vi "SciScan HYPERSCOPE.vi"() -> ()   [LabVIEW 2012]
uses:
  GFG/GFG Translator Wrapper/GFGTranslator_Action.ctl
  GFG/GFG Translator Wrapper/GFGTranslator_Datatype.ctl
  <vilib>/Utility/config.llb/Read Key (String).vi
  <vilib>/Utility/config.llb/NI_LVConfig.lvlib
panel:
  in  "Quit Button":bool
  in  "Imaging Path Reso":bool
  in  "Imaging Path Galvo":bool
  in  "Stimulation Path Galvo":bool
  # "HyperScope Main Control"
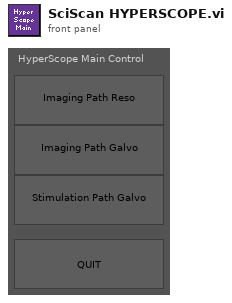
[diagram p1: front panel]
types:
  T1 = enum8{"Enabled", "Disabled", "Disabled and Grayed Out"}
  T2 = typedef "NI_LVConfig.lvlib/Config Data RefNum.ctl" = refnum<k1>
  T3 = enum32{"Invalid", "Standard", "Closed", "Hidden", "Minimized", "Maximized"}
  T4 = typedef "GFGTranslator_Datatype.ctl" = enum16{"String", "Path (String)", "Numeric", "Boolean", "Set_BoolRef (use boolean data)", "Get_Variant", "Get_2DArray (I16)", "Get_Image_2DArray (I16)", "Get_Version (String)", "Get_All GFG variables (String)"}
  T5 = typedef "GFGTranslator_Action.ctl" = enum16{"Get", "Set"}
  T6 = enum16{"Standalone Galvo", "Imaging Galvo", "Photostimulation Galvo"}
  T7 = typedef "GFGTranslator_errors.ctl" = enum16{"Success", "SciScan Not Running", "No Get Method for Selected Datatype", "No Set Method for Selected Datatype", "Variable Not Found", "Unexpected Datatype", "Data Out of Range"}
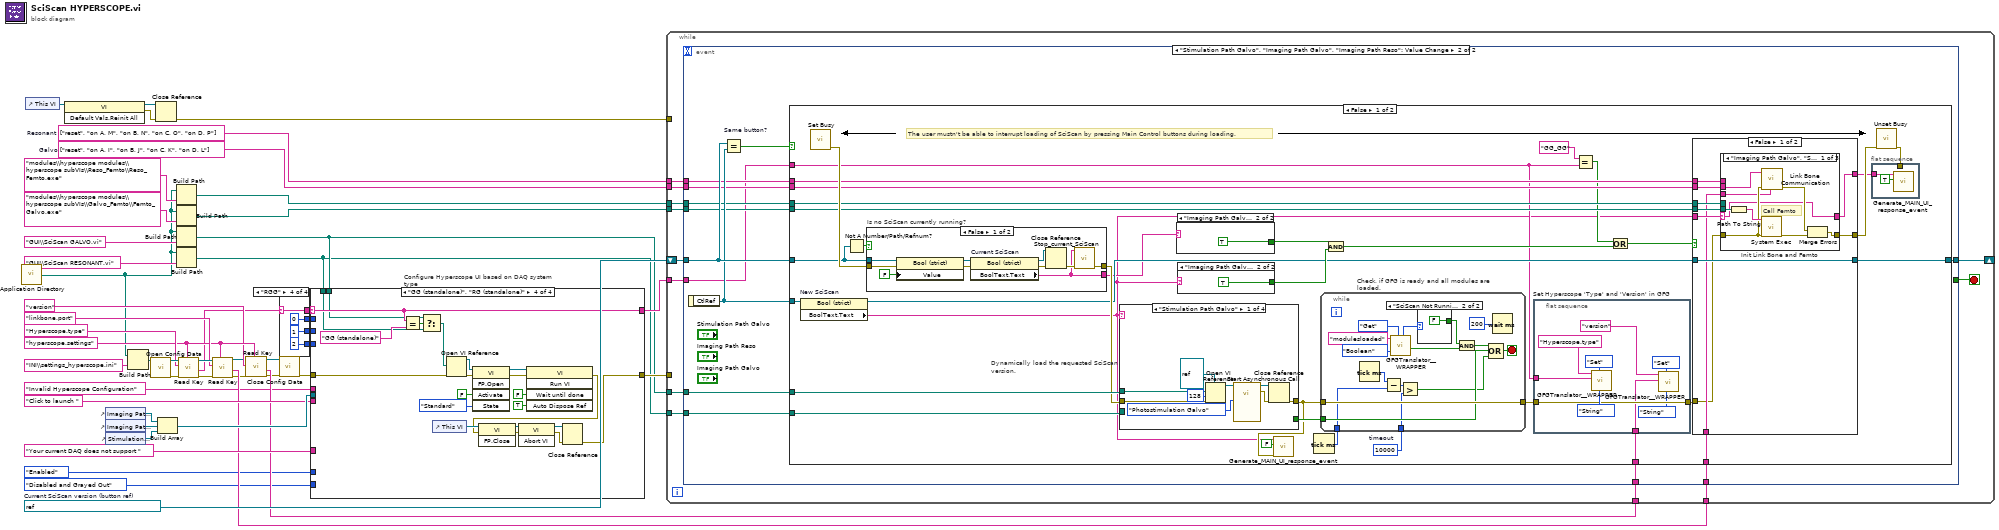
[diagram p0: block diagram]
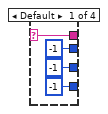
[diagram p2: hidden frame]
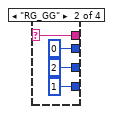
[diagram p3: hidden frame]
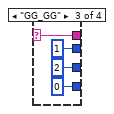
[diagram p4: hidden frame]
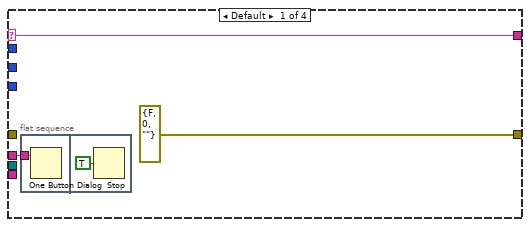
[diagram p5: hidden frame]
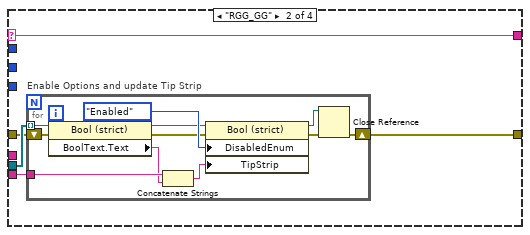
[diagram p6: hidden frame]
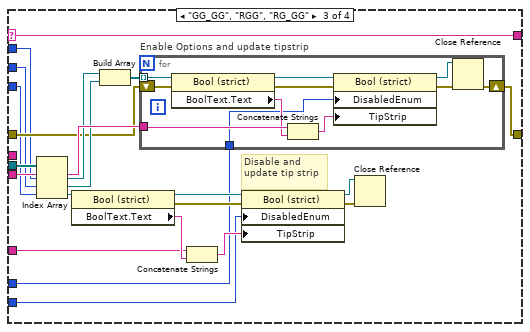
[diagram p7: hidden frame]
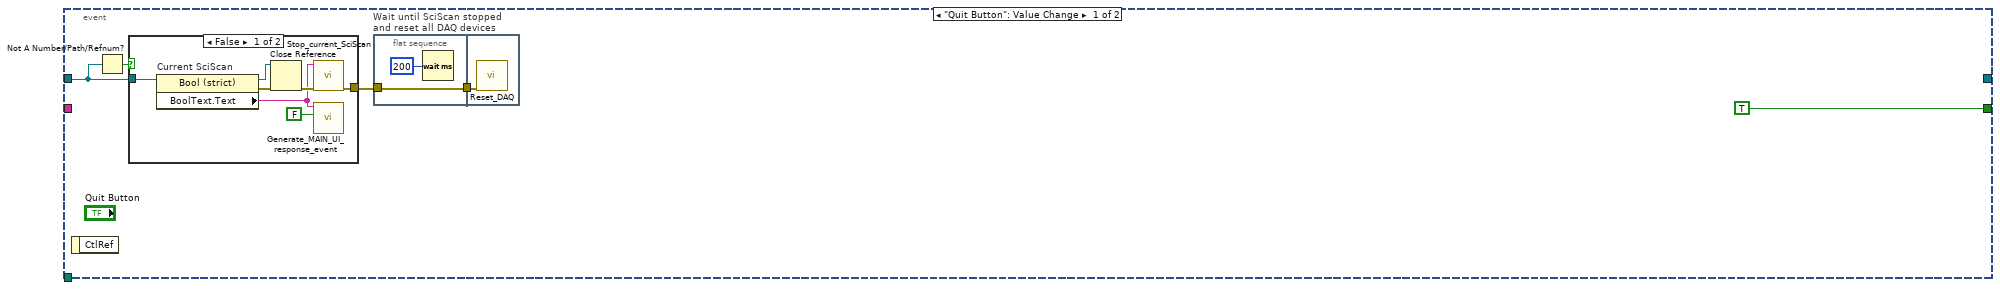
[diagram p8: hidden frame]
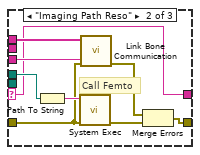
[diagram p12: hidden frame]
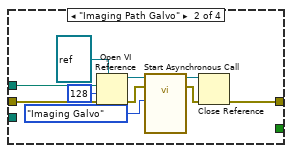
[diagram p15: hidden frame]
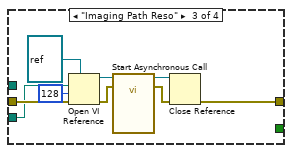
[diagram p16: hidden frame]
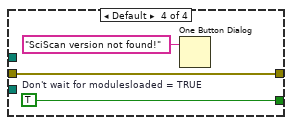
[diagram p17: hidden frame]
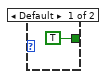
[diagram p18: hidden frame]
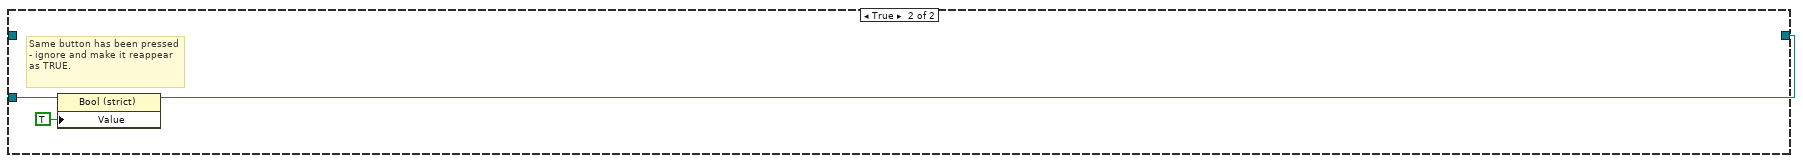
[diagram p20: hidden frame]
diagram:
  w18 = "hyperscope.settings" ("section")
  w40 = string[] ["reset", "on A, I", "on B, J", "on C, K", "on D, L"]  # Galvo
  w41 = string[] ["reset", "on A, M", "on B, N", "on C, O", "on D, P"]  # Resonant
  w42 = refnum<k0> refnum  # Current SciScan version (button ref)
  n1 = call <vilib>:"Application Directory.vi"() -> ("Application Directory"=w3:path)
  n2 = control-ref of="This VI"() -> (w48:refnum<vi>)
  n3 = invoke class="VI" method="Default Vals.Reinit All"(reference=w48) -> (reference out=w46:refnum<vi>, error out=w47:errorcluster)  [unwired: 2 in, 1 out]
  n4 = control-ref of="Imaging Path Reso"() -> (w30:refnum<vi>)
  n5 = control-ref of="Imaging Path Galvo"() -> (w29:refnum<vi>)
  n6 = control-ref of="Stimulation Path Galvo"() -> (w28:refnum<vi>)
  n7 = Build Path(base path=w3, name or relative path="INI\\settings_hyperscope.ini") -> (appended path=w34:path)
  n8 = call <vilib>:"Open Config Data.vi"("configuration file path"=w34) -> ("error out"=w33:errorcluster, "refnum"=w32:T2)  [unwired: 8 in, 1 out]
  n9 = Close Reference(reference=w46, error in (no error)=w47) -> (error out=w45:errorcluster)
  n10 = Build Array(w30, w29, w28) -> (w27:refnum<vi>[])
  n11 = Build Path(base path=w3, name or relative path="modules\\hyperscope modules\\hyperscope subVIs\\Reso_Femto\\Reso_Femto.exe") -> (appended path=w38:path)
  n12 = Build Path(base path=w3, name or relative path="modules\\hyperscope modules\\hyperscope subVIs\\Galvo_Femto\\Femto_Galvo.exe") -> (appended path=w39:path)
  n13 = Build Path(base path=w3, name or relative path="GUI\\SciScan GALVO.vi") -> (appended path=w2:path)
  n14 = Build Path(base path=w3, name or relative path="GUI\\SciScan RESONANT.vi") -> (appended path=w1:path)
  n15 = call-poly <vilib>:"Read Key.vi"("section"=w18, "error in (no error)"=w33, "key"="Hyperscope.type", "refnum"=w32) -> ("error out"=w19:errorcluster, "value"=w9:string, "refnum out"=w22:T2)  [unwired: 4 in, 1 out]
  n16 = call-poly <vilib>:"Read Key.vi"("section"=w18, "error in (no error)"=w19, "key"="linkbone.port", "refnum"=w22) -> ("error out"=w13:errorcluster, "value"=w20:string, "refnum out"=w15:T2)  [unwired: 4 in, 1 out]
  n17 = call-poly <vilib>:"Read Key.vi"("section"=w18, "key"="version", "refnum"=w15) -> ("value"=w16:string, "refnum out"=w14:T2)  [unwired: 5 in, 2 out]
  n18 = case shown="\"RGG\"" w9 {
    selector: w9 -> [w52 w53 w60 w64]
    tunnel: [w52 w53 w60 w64] -> w8
    tunnel: [-1 ("index") 0 ("index") 1 ("index") 0 ("index")] -> w7
    tunnel: [-1 ("index") 2 ("index") 2 ("index") 1 ("index")] -> w6
    tunnel: [-1 ("index") 1 ("index") 0 ("index") 2 ("index")] -> w5
    frame Default {
    }
    frame "RG_GG" {
    }
    frame "GG_GG" {
    }
    frame "RGG" {
    }
  }
  n19 = call <vilib>:"Close Config Data.vi"("error in (no error)"=w13, "refnum"=w14) -> ("error out"=w12:errorcluster)  [unwired: 8 in, 1 out]
  n20 = case "Configure Hyperscope UI based on DAQ system type" shown="\"GG (standalone)\", \"RG (standalone)\"" w8 {
    selector: w8 -> [w67 w71 w92 w135]
    tunnel: w27 -> [_ w74 w97 _]
    tunnel: "Click to launch " ("section") -> [_ w73 w106 _]
    tunnel: [errorcluster {"status"=FALSE, "code"=0, "source"=""} ("error out") w72 w105 w118] -> w25
    tunnel: "Your current DAQ does not support " ("section") -> [_ _ w93 _]
    tunnel: [w67 w71 w92 w135] -> w23
    tunnel: w12 -> [_ w70 w91 w139]
    tunnel: T1."Disabled and Grayed Out" ("Disabled") -> [_ _ w90 _]
    tunnel: T1."Enabled" ("Disabled") -> [_ _ w89 _]
    tunnel: w7 -> [_ _ w88 _]
    tunnel: w6 -> [_ _ w87 _]
    tunnel: w5 -> [_ _ w86 _]
    tunnel: "Invalid Hyperscope Configuration" ("message") -> [w66 _ _ _]
    tunnel: w2 -> [_ _ _ w132]
    tunnel: w1 -> [_ _ _ w131]
    frame Default {
      n21 = flat-sequence {
        tunnel: w66 -> [w68]
        frame #0 {
          n22 = One Button Dialog(message=w68) -> ()  [unwired: 1 in, 1 out]
        }
        frame #1 {
          n23 = Stop(stop? (T)=TRUE) -> ()
        }
      }
    }
    frame "RGG_GG" {
      n24 = for "Enable Options and update Tip Strip" {
        tunnel: w74 -> [w82] mode=indexing
        tunnel: w73 -> [w79]
        shift-right: [w76] -> w72
        shift-left: w70 -> [w75]
        n25 = property class="Bool (strict)"(reference=w82, error in=w75) -> (reference out=w81:refnum<vi>, error out=w80:errorcluster, "BoolText.Text"=w78:string)
        n26 = Concatenate Strings(w79, w78) -> (w77:string)
        n27 = property class="Bool (strict)"(reference=w81, error in=w80, "DisabledEnum"=T1."Enabled" ("Disabled"), "TipStrip"=w77) -> (reference out=w83:refnum<vi>, error out=w84:errorcluster)
        n28 = Close Reference(reference=w83, error in (no error)=w84) -> (error out=w76:errorcluster)
      }
    }
    frame "GG_GG", "RGG", "RG_GG" {
      # "Disable and update tip strip"
      n29 = Index Array(array=w97, index #1=w88, index #2=w87, index #3=w86) -> (element #1=w98:refnum<vi>, element #2=w95:refnum<vi>, element #3=w94:refnum<vi>)
      n30 = property class="Bool (strict)"(reference=w94) -> (reference out=w101:refnum<vi>, error out=w102:errorcluster, "BoolText.Text"=w103:string)  [unwired: 1 in]
      n31 = Build Array(w98, w95) -> (w96:refnum<vi>[])
      n32 = for "Enable Options and update tipstrip" {
        tunnel: w96 -> [w115] mode=indexing
        tunnel: w106 -> [w112]
        shift-right: [w109] -> w105
        shift-left: w91 -> [w108]
        tunnel: w89 -> [w107]
        n33 = property class="Bool (strict)"(reference=w115, error in=w108) -> (reference out=w114:refnum<vi>, error out=w113:errorcluster, "BoolText.Text"=w111:string)
        n34 = Concatenate Strings(w112, w111) -> (w110:string)
        n35 = property class="Bool (strict)"(reference=w114, error in=w113, "DisabledEnum"=w107, "TipStrip"=w110) -> (reference out=w116:refnum<vi>, error out=w117:errorcluster)
        n36 = Close Reference(reference=w116, error in (no error)=w117) -> (error out=w109:errorcluster)
      }
      n37 = Concatenate Strings(w93, w103) -> (w104:string)
      n38 = property class="Bool (strict)"(reference=w101, error in=w102, "DisabledEnum"=w90, "TipStrip"=w104) -> (reference out=w100:refnum<vi>, error out=w99:errorcluster)
      n39 = Close Reference(reference=w100, error in (no error)=w99) -> ()  [unwired: 1 out]
    }
    frame "GG (standalone)", "RG (standalone)" {
      n40 = Equal?(x=w135, y="GG (standalone)" ("name or relative path")) -> (x = y?=w133:bool)
      n41 = Select(t=w132, s=w133, f=w131) -> (s? t:f=w130:path)
      n42 = control-ref of="This VI"() -> (w122:refnum<vi>)
      n43 = Open VI Reference(vi path=w130, error in (no error)=w139) -> (vi reference=w128:refnum<vi>, error out=w127:errorcluster)  [unwired: 4 in]
      n44 = invoke class="VI" method="FP.Open"(reference=w128, error in=w127, "Activate"=FALSE ("Activate?"), "State"=T3."Standard") -> (reference out=w124:refnum<vi>, error out=w123:errorcluster)  [unwired: 1 in, 3 out]
      n45 = invoke class="VI" method="Run VI"(reference=w124, error in=w123, "Wait until done"=FALSE ("Wait Until Done"), "Auto Dispose Ref"=TRUE ("Auto Dispose Reference")) -> (error out=w121:errorcluster)  [unwired: 1 in, 4 out]
      n46 = invoke class="VI" method="FP.Close"(reference=w122, error in=w121) -> (reference out=w119:refnum<vi>, error out=w120:errorcluster)  [unwired: 1 in, 1 out]
      n47 = invoke class="VI" method="Abort VI"(reference=w119, error in=w120) -> (reference out=w137:refnum<vi>, error out=w136:errorcluster)  [unwired: 1 in, 1 out]
      n48 = Close Reference(reference=w137, error in (no error)=w136) -> (error out=w118:errorcluster)
    }
  }
  n49 = while {
    tunnel: w45 -> [_]
    tunnel: w2 -> [w150]
    tunnel: w1 -> [w149]
    shift-right: [w148] -> _
    shift-left: w42 -> [w147]
    tunnel: w41 -> [w146]
    tunnel: w40 -> [w145]
    tunnel: w38 -> [w144]
    tunnel: w39 -> [w143]
    tunnel: w25 -> [_]
    tunnel: w23 -> [w142]
    tunnel: w20 -> [w141]
    tunnel: w16 -> [w140]
    stop <- w151 stop-if-true
    n50 = event shown="[1] \"Stimulation Path Galvo\", \"Imaging Path Galvo\", \"Imaging Path Reso\": Value Change" {
      selector: _ -> [_ _]
      dyn-events: _ -> [_ _]
      timeout: _ -> [_ _]
      tunnel: [TRUE _] -> w151
      tunnel: w150 -> [_ w179]
      tunnel: w149 -> [_ w174]
      tunnel: [_ w176] -> w148
      tunnel: w147 -> [w155 w178]
      tunnel: w146 -> [_ w173]
      tunnel: w145 -> [_ w172]
      tunnel: w144 -> [_ w171]
      tunnel: w143 -> [_ w170]
      tunnel: w142 -> [_ w168]
      tunnel: w141 -> [_ w169]
      tunnel: w140 -> [_ w167]
      event "Quit Button": Value Change {
        n51 = event-data() -> ()  [unwired: 1 in, 1 out]
        n52 = Not A Number/Path/Refnum?(number/path/refnum=w155) -> (NaN/Path/Refnum?=w154:bool)
        n53 = case shown="False" w154 {
          tunnel: w155 -> [w163 _]
          tunnel: [w162 _] -> w153
          frame False {
            n54 = property on="Current SciScan" class="Bool (strict)"(reference=w163) -> (reference out=w166:refnum<vi>, error out=w165:errorcluster, "BoolText.Text"=w160:string)  [unwired: 1 in]
            n55 = Close Reference(reference=w166, error in (no error)=w165) -> (error out=w164:errorcluster)
            n56 = call "Stop_current_SciScan.vi"("error in (no error)"=w164, "Current SciScan"=w160) -> ("error out"=w162:errorcluster)  [unwired: 9 in]
            n57 = call "Generate_MAIN_UI_response_event.vi"("Responsive? (F)"=FALSE, "System Type"=w160) -> ()  [unwired: 9 in, 1 out]
          }
          frame True {
          }
        }
        n58 = flat-sequence "Wait until SciScan stopped\nand reset all DAQ devices" {
          tunnel: w153 -> [w158]
          tunnel: [w158] -> w152
          tunnel: w152 -> [w159]
          frame #0 {
            n59 = Wait (ms)(milliseconds to wait=u32 200) -> ()  [unwired: 1 out]
          }
          frame #1 {
            n60 = call "Reset_DAQ.vi"("error in (no error)"=w159) -> ()  [unwired: 10 in, 1 out]
          }
        }
      }
      event "Stimulation Path Galvo", "Imaging Path Galvo", "Imaging Path Reso": Value Change {
        n61 = event-data() -> ("CtlRef"=w175:refnum<vi>)  [unwired: 1 in]
        n62 = Equal? "Same button?"(x=w178, y=w175) -> (x = y?=w177:bool)
        n63 = case shown="False" w177 {
          tunnel: w179 -> [w213 _]
          tunnel: w178 -> [w210 _]
          tunnel: [w197 w320] -> w176
          tunnel: w175 -> [w209 w322]
          tunnel: w174 -> [w208 _]
          tunnel: w173 -> [w206 _]
          tunnel: w172 -> [w205 _]
          tunnel: w171 -> [w204 _]
          tunnel: w170 -> [w203 _]
          tunnel: w169 -> [w195 _]
          tunnel: w168 -> [w188 _]
          tunnel: w167 -> [w187 _]
          frame False {
            w185 = u32 10000  # timeout
            # "The user mustn't be able to interrupt loading of SciScan by pressing Main Control buttons during loading."
            n64 = property on="New SciScan" class="Bool (strict)"(reference=w209) -> (reference out=w198:refnum<vi>, "BoolText.Text"=w180:string)  [unwired: 1 in, 1 out]
            n65 = call <vilib>:"Set Busy.vi"() -> ("error out"=w211:errorcluster)  [unwired: 10 in, 1 out]
            n66 = Not A Number/Path/Refnum?(number/path/refnum=w210) -> (NaN/Path/Refnum?=w212:bool)
            n67 = case "Is no SciScan currently running?" shown="False" w212 {
              tunnel: [w315 w319] -> w202
              tunnel: w211 -> [w316 w319]
              tunnel: w210 -> [w317 _]
              tunnel: [w309 _] -> w196
              frame False {
                n68 = property class="Bool (strict)"(reference=w317, error in=w316, "Value"=FALSE) -> (reference out=w312:refnum<vi>, error out=w313:errorcluster)
                n69 = property on="Current SciScan" class="Bool (strict)"(reference=w312, error in=w313) -> (reference out=w311:refnum<vi>, error out=w310:errorcluster, "BoolText.Text"=w309:string)
                n70 = Close Reference(reference=w311, error in (no error)=w310) -> (error out=w314:errorcluster)
                n71 = call "Stop_current_SciScan.vi"("error in (no error)"=w314, "Current SciScan"=w309) -> ("error out"=w315:errorcluster)  [unwired: 9 in]
              }
              frame True {
              }
            }
            n72 = case "Dynamically load the requested SciScan version." shown="\"Stimulation Path Galvo\"" w180 {
              tunnel: w213 -> [w268 w278 _ _]
              tunnel: [w260 w270 w279 w290] -> w181
              tunnel: w202 -> [w263 w273 w284 w290]
              tunnel: w208 -> [_ _ w282 _]
              tunnel: [_ _ _ w288] -> w207
              frame "Stimulation Path Galvo" {
                n73 = Open VI Reference(type specifier VI Refnum (for type only)=refnum<vi> refnum ("reference"), vi path=w268, options=128, error in (no error)=w263) -> (vi reference=w265:refnum<vi>)  [unwired: 2 in, 1 out]
                n74 = call-by-ref "Start Asynchronous Call"(reference=w265, "System type (Default - Standalone)"=T6."Photostimulation Galvo") -> (reference out=w261:refnum<vi>, error out=w262:errorcluster)  [unwired: 12 in]
                n75 = Close Reference(reference=w261, error in (no error)=w262) -> (error out=w260:errorcluster)
              }
              frame "Imaging Path Galvo" {
                n76 = Open VI Reference(type specifier VI Refnum (for type only)=refnum<vi> refnum ("reference"), vi path=w278, options=128, error in (no error)=w273) -> (vi reference=w275:refnum<vi>, error out=w269:errorcluster)  [unwired: 2 in]
                n77 = call-by-ref "Start Asynchronous Call"(reference=w275, error in=w269, "System type (Default - Standalone)"=T6."Imaging Galvo") -> (reference out=w271:refnum<vi>, error out=w272:errorcluster)  [unwired: 11 in]
                n78 = Close Reference(reference=w271, error in (no error)=w272) -> (error out=w270:errorcluster)
              }
              frame "Imaging Path Reso" {
                n79 = Open VI Reference(type specifier VI Refnum (for type only)=refnum<vi> refnum, vi path=w282, options=128, error in (no error)=w284) -> (vi reference=w285:refnum<vi>, error out=w283:errorcluster)  [unwired: 2 in]
                n80 = call-by-ref "Start Asynchronous Call"(reference=w285, error in=w283) -> (reference out=w281:refnum<vi>, error out=w280:errorcluster)  [unwired: 12 in]
                n81 = Close Reference(reference=w281, error in (no error)=w280) -> (error out=w279:errorcluster)
              }
              frame Default {
                w288 = TRUE  # Don't wait for modulesloaded = TRUE
                n82 = One Button Dialog(message="SciScan version not found!") -> ()  [unwired: 1 in, 1 out]
              }
            }
            n83 = case shown="\"Imaging Path Galvo\", \"Stimulation Path Galvo\"" w196 {
              tunnel: [_ TRUE] -> w200
              frame "False", Default {
              }
              frame "Imaging Path Galvo", "Stimulation Path Galvo" {
              }
            }
            n84 = case shown="\"Imaging Path Galvo\", \"Stimulation Path Galvo\"" w180 {
              tunnel: [_ TRUE] -> w199
              frame "False", Default {
              }
              frame "Imaging Path Galvo", "Stimulation Path Galvo" {
              }
            }
            n85 = call "Generate_MAIN_UI_response_event.vi"("error in (no error)"=w181, "Responsive? (F)"=FALSE, "System Type"=w180) -> ()  [unwired: 8 in, 1 out]
            n86 = Tick Count (ms)() -> (millisecond timer value=w186:u32)
            n87 = while "Check, if GFG is ready and all modules are loaded." {
              tunnel: w181 -> [w306]
              tunnel: [w306] -> w190
              tunnel: w207 -> [w302]
              tunnel: w186 -> [w293]
              tunnel: w185 -> [w292]
              stop <- w303 stop-if-true
              n88 = Tick Count (ms)() -> (millisecond timer value=w294:u32)
              n89 = Subtract(x=w294, y=w293) -> (x-y=w295:u32)
              n90 = call "GFGTranslator__WRAPPER.vi"("GFGTranslator Datatype"=GFGTranslator_Datatype."Boolean", "GFG Translator Action"=GFGTranslator_Action."Get", "GFG Variable Name"="modulesloaded" ("Variable Name in")) -> ("Boolean_Output"=w299:bool, "Status Output"=w298:T7)  [unwired: 3 in, 4 out]
              n91 = Greater?(x=w295, y=w292) -> (0:w291:bool)
              n92 = case shown="\"SciScan Not Running\"" w298 {
                tunnel: [TRUE FALSE] -> w297
                frame Default {
                }
                frame "SciScan Not Running" {
                }
              }
              n93 = And(x=w297, y=w299) -> (x .and. y?=w304:bool)
              n94 = Compound Arithmetic op=OR(w304, w302, w291) -> (w303:bool)
              n95 = Wait (ms)(milliseconds to wait=u32 200) -> ()  [unwired: 1 out]
            }
            n96 = And(x=w200, y=w199) -> (x .and. y?=w192:bool)
            n97 = flat-sequence "Set Hyperscope 'Type' and 'Version' in GFG" {
              tunnel: w190 -> [w221]
              tunnel: [w221] -> w189
              tunnel: w188 -> [w220]
              tunnel: w187 -> [w216]
              frame #0 {
                n98 = call "GFGTranslator__WRAPPER.vi"("GFGTranslator Datatype"=GFGTranslator_Datatype."String", "GFG Translator Action"=GFGTranslator_Action."Set", "String_Input"=w220, "GFG Variable Name"="Hyperscope.type" ("Variable Name in")) -> ()  [unwired: 2 in, 6 out]
                n99 = call "GFGTranslator__WRAPPER.vi"("GFGTranslator Datatype"=GFGTranslator_Datatype."String", "GFG Translator Action"=GFGTranslator_Action."Set", "String_Input"=w216, "GFG Variable Name"="version" ("Variable Name in")) -> ()  [unwired: 2 in, 6 out]
              }
            }
            n100 = Equal?(x="GG_GG", y=w188) -> (x = y?=w191:bool)
            n101 = Or(x=w191, y=w192) -> (x .or. y?=w193:bool)
            n102 = case shown="False" w193 {
              tunnel: w180 -> [w236 w257]
              tunnel: w206 -> [w235 _]
              tunnel: w205 -> [w234 _]
              tunnel: w204 -> [w233 _]
              tunnel: w203 -> [w232 _]
              tunnel: w189 -> [w228 w259]
              tunnel: [w231 w259] -> w201
              tunnel: w198 -> [w230 w258]
              tunnel: [w230 w258] -> w197
              tunnel: w195 -> [w229 _]
              tunnel: [w227 w257] -> w183
              frame False {
                n103 = case "Init Link Bone and Femto" shown="\"Imaging Path Galvo\", \"Stimulation Path Galvo\"" w236 {
                  selector: w236 -> [w237 w246 w255]
                  tunnel: w235 -> [_ w254 _]
                  tunnel: w234 -> [w243 _ _]
                  tunnel: w233 -> [_ w253 _]
                  tunnel: w232 -> [w245 _ _]
                  tunnel: w228 -> [w242 w247 w256]
                  tunnel: [w239 w249 w256] -> w231
                  tunnel: w229 -> [w238 w248 _]
                  tunnel: [w237 w246 w255] -> w227
                  frame "Imaging Path Galvo", "Stimulation Path Galvo" {
                    # "Call Femto"
                    n104 = Path To String(path=w245) -> (string=w244:string)
                    n105 = call <vilib>:"System Exec.vi"("error in (no error)"=w242, "command line"=w244) -> ("error out"=w240:errorcluster)  [unwired: 6 in, 3 out]
                    n106 = call "Link Bone Communication.vi"("VISA resource name"=w238, "error in"=w242, "Commands"=w243) -> ("error out"=w241:errorcluster)  [unwired: 8 in]
                    n107 = Merge Errors(w241, w240) -> (w239:errorcluster)
                  }
                  frame "Imaging Path Reso" {
                    # "Call Femto"
                    n108 = Path To String(path=w253) -> (string=w252:string)
                    n109 = call <vilib>:"System Exec.vi"("error in (no error)"=w247, "command line"=w252) -> ("error out"=w251:errorcluster)  [unwired: 6 in, 3 out]
                    n110 = call "Link Bone Communication.vi"("VISA resource name"=w248, "error in"=w247, "Commands"=w254) -> ("error out"=w250:errorcluster)  [unwired: 8 in]
                    n111 = Merge Errors(w250, w251) -> (w249:errorcluster)
                  }
                  frame Default {
                  }
                }
              }
              frame True {
              }
            }
            n112 = flat-sequence {
              tunnel: w184 -> [_]
              tunnel: w183 -> [w215]
              frame #0 {
                n113 = call "Generate_MAIN_UI_response_event.vi"("Responsive? (F)"=TRUE, "System Type"=w215) -> ()  [unwired: 9 in, 1 out]
              }
            }
            n114 = call <vilib>:"Unset Busy.vi"("error in (no error)"=w201) -> ("error out"=w184:errorcluster)  [unwired: 10 in]
          }
          frame True {
            # "Same button has been pressed - ignore and make it reappear as TRUE."
            n115 = property class="Bool (strict)"(reference=w322, "Value"=TRUE) -> (reference out=w320:refnum<vi>)  [unwired: 1 in, 1 out]
          }
        }
      }
    }
  }
